vi "Do.vi"(8 "error in (no error)":errorcluster, 10 "Actor in":refnum<class "Actor.lvclass">, 11 "SetPrivileges Msg":refnum<class "SetPrivileges Msg.lvclass">) -> (0 "error out":errorcluster, 2 "Actor out":refnum<class "Actor.lvclass">)   [LabVIEW 2019, in "TestBench.lvlib" / "SetPrivileges Msg.lvclass"]
doc: "This VI delivers the message to the actor by calling the appropriate method(s) on the actor."
uses:
  SetPrivileges Msg.lvclass
  C:/Program Files (x86)/National Instruments/LabVIEW 2019/vi.lib/NI/Event Source Actor/Event Source/Event Source Messages/Event Generated Msg/Event Generated Msg.lvclass
  <vilib>/ActorFramework/Actor/Actor.lvclass
  TestBench/TestBench.lvclass
  C:/Program Files (x86)/National Instruments/LabVIEW 2019/vi.lib/ActorFramework/Actor/Actor.lvclass
  UserManagement/UserManagement/UserInfo.lvclass
  <vilib>/NI/Event Source Actor/Event Source/Event Source Messages/Event Generated Msg/Event Generated Msg.lvclass/Event Generated Msg.ctl
  <vilib>/NI/Event Source Actor/Event Source/Event Source Messages/Event Generated Msg/Event Generated Msg.lvclass
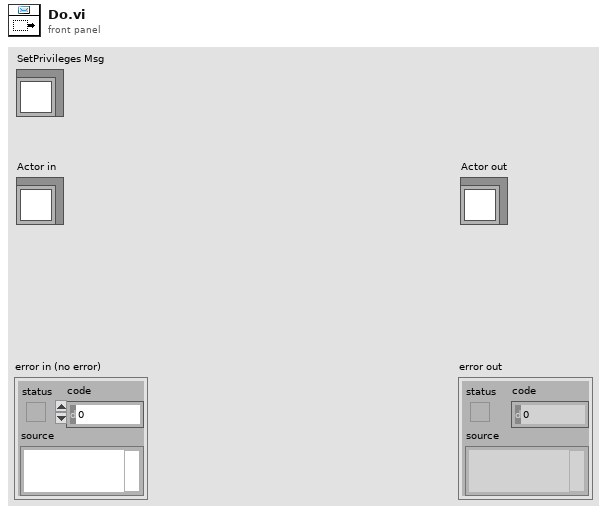
[diagram p1: front panel]
types:
  T1 = typedef "UserManagement.lvlib/UserManagement.lvclass/UserInfo.ctl" = cluster{"Privileges":T2, "UserName":string}
  T2 = typedef "UserManagement.lvlib/UserManagement.lvclass/Permission.ctl" = enum16{"Engineer", "Technical", "Operator"}
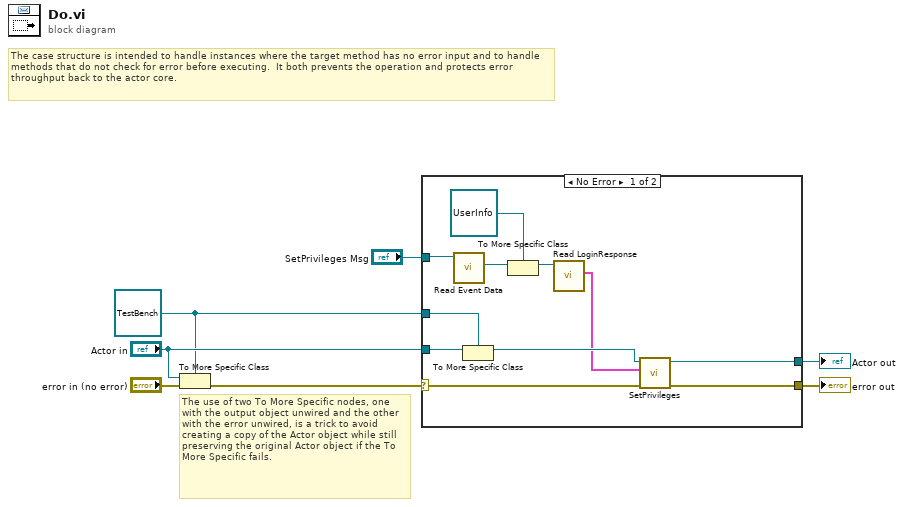
[diagram p0: block diagram]
diagram:
  w2 = refnum<class "TestBench.lvclass"> refnum ("Actor in")
  # "The use of two To More Specific nodes, one with the output object unwired and the other with the error unwired, is a trick to avoid creating a copy of the Actor object while still preserving the original Actor object if the To More Specific fails."
  # "The case structure is intended to handle instances where the target method has no error input and to handle methods that do not check for error before executing.  It both prevents the operation and protects error throughput back to the actor core."
  n1 = To More Specific Class(target class=w2, reference="Actor in", error in="error in (no error)") -> (error out=w6:errorcluster)  [unwired: 1 out]
  n2 = case shown="No Error" w6 {
    selector: w6 -> [w16 w20]
    tunnel: [w18 w20] -> w5
    tunnel: [w17 w19] -> w4
    tunnel: "Actor in" -> [w15 w19]
    tunnel: w2 -> [w14 _]
    tunnel: "SetPrivileges Msg" -> [w12 _]
    frame No Error {
      n3 = call <vilib>:"Read Event Data.vi"("Event Generated Msg"=w12) -> ("Event Data"=w11:refnum<class "Event.lvclass">)  [unwired: 10 in]
      n4 = To More Specific Class(target class=w14, reference=w15) -> (specific class reference=w13:refnum<class "TestBench.lvclass">)  [unwired: 1 in, 1 out]
      n5 = To More Specific Class(target class=refnum<class "UserInfo.lvclass"> refnum ("UserManagement.lvlib:UserInfo.lvclass"), reference=w11) -> (specific class reference=w9:refnum<class "UserInfo.lvclass">)  [unwired: 1 in, 1 out]
      n6 = call-dynamic "Read LoginResponse.vi"("UserInfo in"=w9) -> ("LoginResponse"=w8:cluster{"UserInfo":T1, "PassWordExists？":bool})  [unwired: 8 in, 2 out]
      n7 = call-dynamic "SetPrivileges.vi"("error in (no error)"=w16, "LoginResponse"=w8, "TestBench in"=w13) -> ("error out"=w18:errorcluster, "TestBench out"=w17:refnum<class "TestBench.lvclass">)  [unwired: 7 in]
    }
    frame Error {
      # "If type check fails, pass the original object out again."
    }
  }
  "error out" <- w5
  "Actor out" <- w4
